vi "Prepare Elevation Grid.vi"(6 "Current Location Identifier (S)":string="S", 7 "Best Signal Location Identifier (E)":string="E", 9 "Plain Elevation Grid":string="Sabqponm\nabcryxxl\naccszExk\nacctuvwj\nabdefghi") -> (0 "Current Location":cdb, 1 "Best Signal Location":cdb, 4 "Elevation Grid":string[][](array[string]), 5 "Elevation Grid Numeric":i32[][](array[numeric]))   [LabVIEW 2020, in "AoC 2022.lvlib"]
uses:
  AoC 2022.lvlib
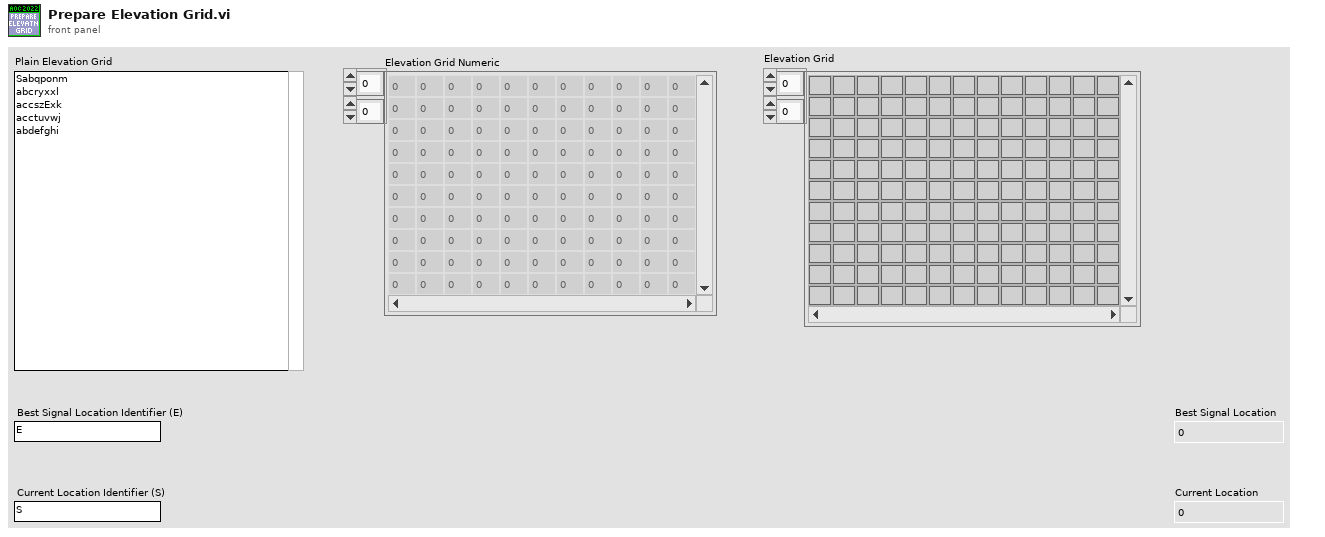
[diagram p1: front panel]
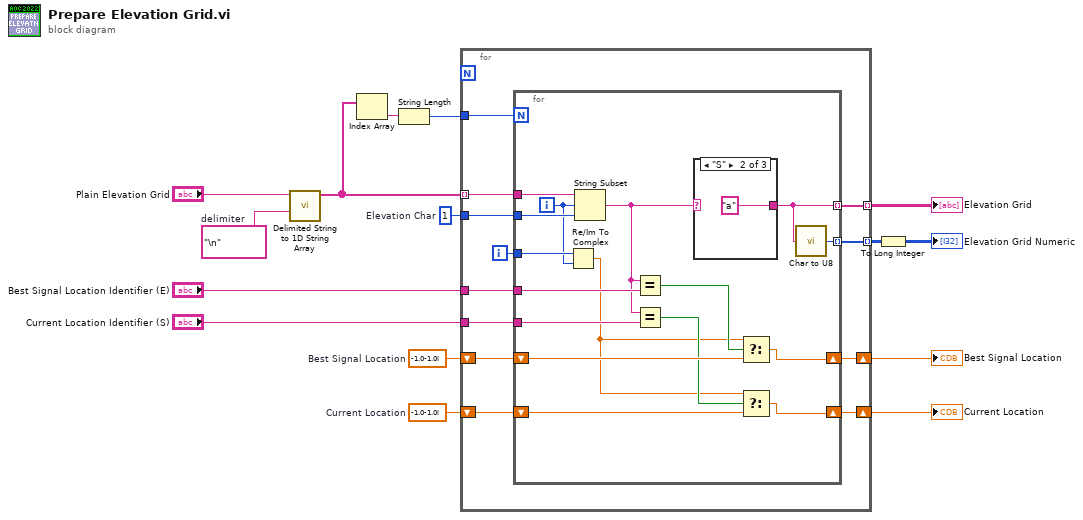
[diagram p0: block diagram]
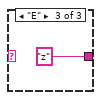
[diagram p3: hidden frame]
diagram:
  w4 = "\n"  # delimiter
  w12 = cdb -1.0-1.0i  # Current Location
  w11 = cdb -1.0-1.0i  # Best Signal Location
  w8 = 1  # Elevation Char
  n1 = call <vilib>:"Delimited String to 1D String Array.vi"("delimiter"=w4, "delimited string"="Plain Elevation Grid") -> ("string array"=w3:string[])  [unwired: 9 in]
  n2 = Index Array(array=w3) -> (element=w6:string)  [unwired: 1 in]
  n3 = String Length(string=w6) -> (length=w7:i32)
  n4 = for {
    tunnel: w3 -> [w27] mode=indexing
    tunnel: w7 -> [w26]
    tunnel: w8 -> [w25]
    tunnel: [w24] -> w13 mode=indexing
    tunnel: "Best Signal Location Identifier (E)" -> [w23]
    tunnel: "Current Location Identifier (S)" -> [w22]
    shift-right: [w18] -> w14
    shift-left: w11 -> [w21]
    shift-right: [w17] -> w15
    shift-left: w12 -> [w20]
    tunnel: [w16] -> w2 mode=indexing
    i -> [w19]
    n5 = for {
      N: w26 -> [_]
      tunnel: w27 -> [w43]
      tunnel: w25 -> [w42]
      tunnel: [w29] -> w24 mode=indexing
      tunnel: w23 -> [w41]
      tunnel: w22 -> [w40]
      shift-right: [w35] -> w18
      shift-left: w21 -> [w36]
      shift-right: [w33] -> w17
      shift-left: w20 -> [w34]
      tunnel: w19 -> [w38]
      tunnel: [w28] -> w16 mode=indexing
      i -> [w37]
      n6 = Re/Im To Complex(1:w37, 2:w38) -> (0:w31:cdb)
      n7 = String Subset(string=w43, offset (0)=w37, length (rest)=w42) -> (substring=w30:string)
      n8 = Equal?(x=w30, y=w41) -> (x = y?=w39:bool)
      n9 = Equal?(x=w30, y=w40) -> (x = y?=w32:bool)
      n10 = case shown="\"S\"" w30 {
        selector: w30 -> [w44 _ _]
        tunnel: [w44 "a" "z"] -> w29
        frame Default {
        }
        frame "S" {
        }
        frame "E" {
        }
      }
      n11 = Select(t=w31, s=w39, f=w36) -> (s? t:f=w35:cdb)
      n12 = Select(t=w31, s=w32, f=w34) -> (s? t:f=w33:cdb)
      n13 = call "Char to U8.vi"("Char"=w29) -> ("U8"=w28:u8)
    }
  }
  "Current Location" <- w15
  "Best Signal Location" <- w14
  "Elevation Grid" <- w13
  n14 = To Long Integer(number=w2) -> (32bit integer=→"Elevation Grid Numeric":i32[][])
